vi "Filter Categories.vi"(8 "error in (no error)":errorcluster, 10 "String Input":string, 11 "Budgetizer in":refnum<class "Budgetizer.lvclass">) -> (0 "error out":errorcluster, 2 "Matching Categories":refnum<class "Category.lvclass">[](array[class]), 3 "Budgetizer out":refnum<class "Budgetizer.lvclass">)   [LabVIEW 2018, in "Budgetizer.lvclass"]
uses:
  Budgetizer.lvclass
  Category/Category.lvclass
  Budgetizer.lvclass/Budgetizer.ctl
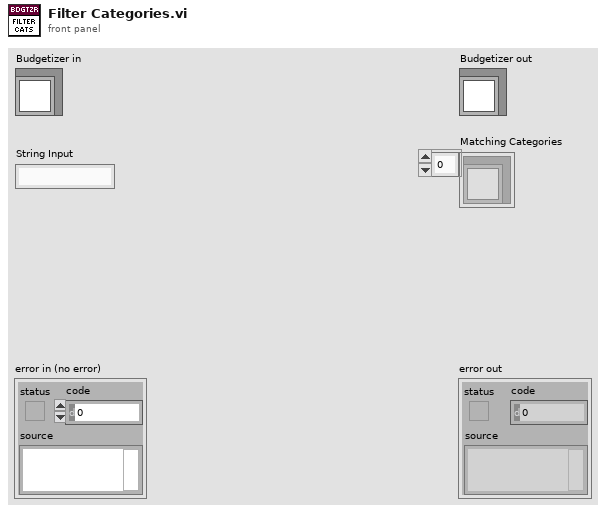
[diagram p1: front panel]
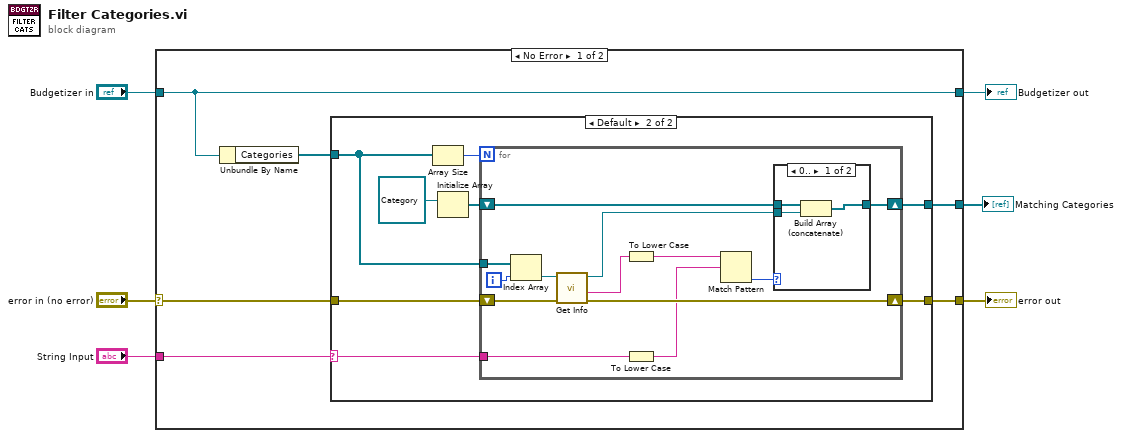
[diagram p0: block diagram]
diagram:
  n1 = case shown="No Error" "error in (no error)" {
    selector: "error in (no error)" -> [w10 w41]
    tunnel: [w9 w41] -> w5
    tunnel: [w12 w40] -> w3
    tunnel: "Budgetizer in" -> [w12 w40]
    tunnel: "String Input" -> [w7 _]
    tunnel: [w8 _] -> w1
    frame No Error {
      n2 = Unbundle By Name(w12) -> ("Categories"=w11:refnum<class "Category.lvclass">[])
      n3 = case shown="Default" w7 {
        selector: w7 -> [_ w17]
        tunnel: w11 -> [w14 w21]
        tunnel: w10 -> [w13 w20]
        tunnel: [w13 w19] -> w9
        tunnel: [w14 w18] -> w8
        frame "" {
        }
        frame Default {
          n4 = Array Size(array=w21) -> (size(s)=w22:i32)
          n5 = Initialize Array(refnum<class "Category.lvclass"> refnum ("element")) -> (w15:refnum<class "Category.lvclass">[])  [unwired: 1 in]
          n6 = for {
            N: w22 -> [_]
            tunnel: w17 -> [w28]
            tunnel: w21 -> [w34]
            shift-right: [w32] -> w19
            shift-left: w20 -> [w33]
            shift-right: [w30] -> w18
            shift-left: w15 -> [w31]
            i -> [w35]
            n7 = Index Array(array=w34, index=w35) -> (element=w29:refnum<class "Category.lvclass">)
            n8 = call "Get Info.vi"("error in (no error)"=w33, "Category in"=w29) -> ("error out"=w32:errorcluster, "Name"=w24:string, "Category out"=w23:refnum<class "Category.lvclass">)  [unwired: 6 in, 1 out]
            n9 = To Lower Case(string=w24) -> (all lower case string=w27:string)
            n10 = To Lower Case(string=w28) -> (all lower case string=w25:string)
            n11 = Match Pattern(string=w27, regular expression=w25) -> (offset past match=w26:i32)  [unwired: 1 in, 3 out]
            n12 = case shown="0.." w26 {
              tunnel: [w38 w39] -> w30
              tunnel: w31 -> [w37 w39]
              tunnel: w23 -> [w36 _]
              frame 0.. {
                n13 = Build Array (concatenate)(w37, w36) -> (w38:refnum<class "Category.lvclass">[])
              }
              frame Default {
              }
            }
          }
        }
      }
    }
    frame Error {
    }
  }
  "error out" <- w5
  "Budgetizer out" <- w3
  "Matching Categories" <- w1
